vi "Test_NewProtocolEntry.vi"() -> ()   [LabVIEW 2014]
uses:
  controls/ProtocolT.ctl
  controls/ProtocolEntry.ctl
panel:
  out "MyProtocol":T1 {"Zeitstempel" format=" %<%X %x>T"}
  in  "Stopp":bool
  in  "AddEntry":bool
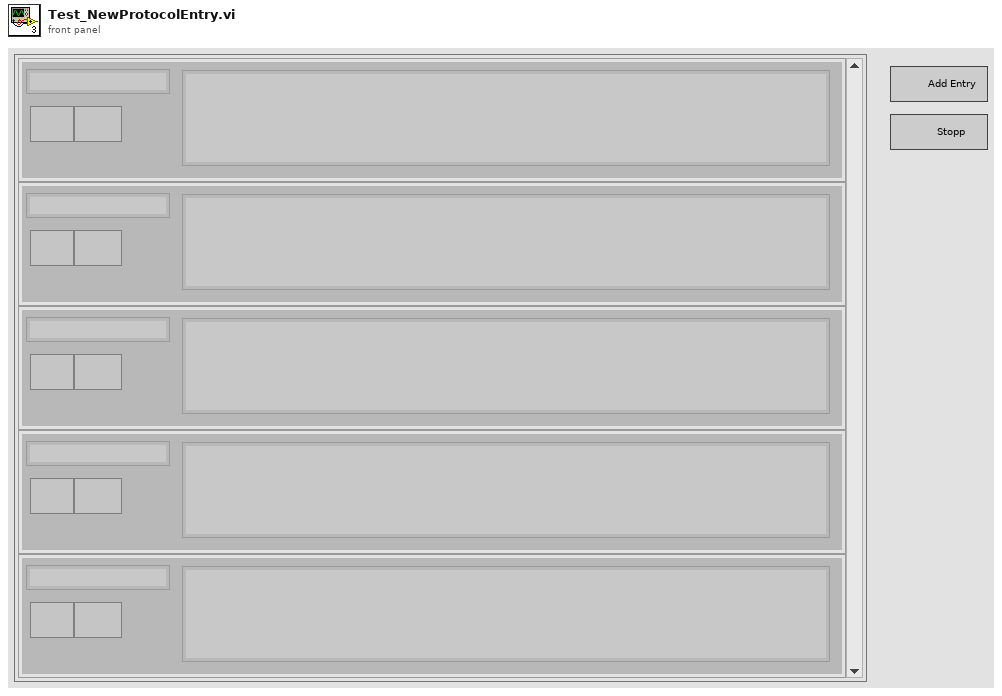
[diagram p1: front panel]
types:
  T1 = typedef "ProtocolT.ctl" = T2[]
  T2 = typedef "ProtocolEntry.ctl" = cluster{"Zeitstempel":timestamp, "String":string, "Abbrechen-Schaltfläche":bool, "Optionen-Schaltfläche":bool}
  T3 = cluster{"AddEntry":refnum<vi>, "Stopp":refnum<vi>}
  T4 = cluster{cluster{"MyProtocol":refnum<vi>}, cluster{"AddEntry":refnum<vi>, "Stopp":refnum<vi>}}
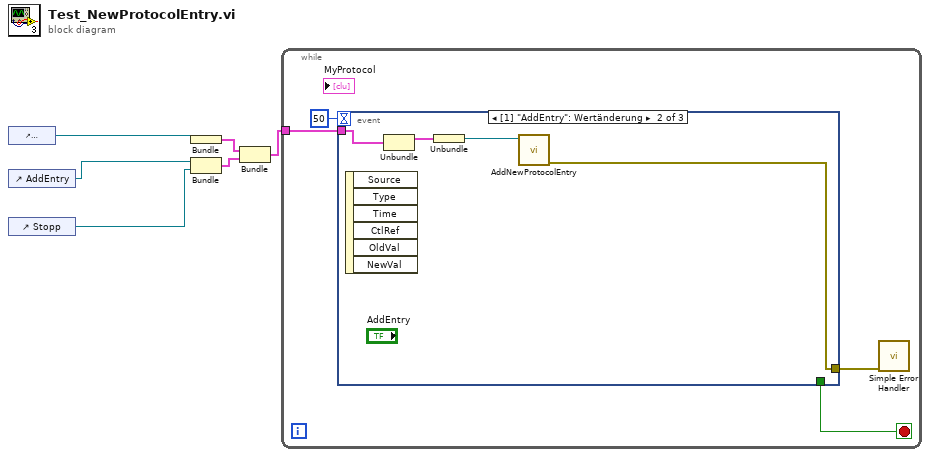
[diagram p0: block diagram]
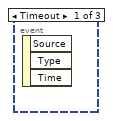
[diagram p2: hidden frame]
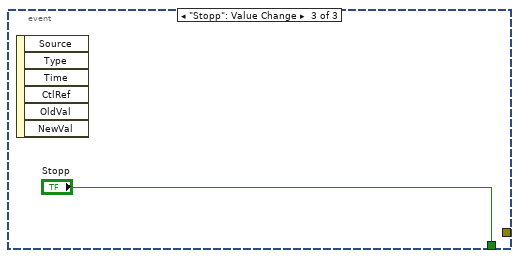
[diagram p3: hidden frame]
diagram:
  n1 = control-ref of="MyProtocol"() -> (w2:refnum<vi>)
  n2 = control-ref of="AddEntry"() -> (w6:refnum<vi>)
  n3 = control-ref of="Stopp"() -> (w1:refnum<vi>)
  n4 = Bundle("MyProtocol"=w2) -> (w5:cluster{"MyProtocol":refnum<vi>})  [unwired: 1 in]
  n5 = Bundle("AddEntry"=w6, "Stopp"=w1) -> (w4:T3)  [unwired: 1 in]
  n6 = Bundle(w5, w4) -> (w3:T4)  [unwired: 1 in]
  n7 = while {
    tunnel: w3 -> [w10]
    stop <- w9 stop-if-true
    n8 = event shown="[1] \"AddEntry\": Wertänderung" {
      selector: _ -> [_ _ _]
      dyn-events: _ -> [_ _ _]
      timeout: 50 -> [_ _ _]
      tunnel: w10 -> [_ w14 _]
      tunnel: [_ _ "Stopp"] -> w9
      tunnel: [_ w11 _] -> w7
      event Timeout {
        n9 = event-data() -> ()  [unwired: 1 in, 3 out]
      }
      event "AddEntry": Value Change {
        n10 = event-data() -> ()  [unwired: 1 in, 6 out]
        n11 = Unbundle(w14) -> (w13:cluster{"MyProtocol":refnum<vi>})  [unwired: 1 out]
        n12 = Unbundle(w13) -> ("MyProtocol"=w12:refnum<vi>)
        n13 = call "AddNewProtocolEntry.vi"("Array (Eingang)"=w12) -> ("Fehler (Ausgang)"=w11:errorcluster)  [unwired: 9 in, 1 out]
      }
      event "Stopp": Value Change {
        n14 = event-data() -> ()  [unwired: 1 in, 6 out]
      }
    }
    n15 = call <vilib>:"Simple Error Handler.vi"("error in (no error)"=w7) -> ()  [unwired: 4 in, 5 out]
  }
